vi "Read growables.vi"(9 "Diagram in":refnum<class "Diagram.lvclass">) -> (3 "Diagram out":refnum<class "Diagram.lvclass">, 4 "growables":refnum<class "GrowableFunction.lvclass">[](array[class]))   [LabVIEW 2014, in "Diagram.lvclass"]
uses:
  Diagram.lvclass
  GrowableFunction/GrowableFunction.lvclass
  Diagram.lvclass/Diagram.ctl
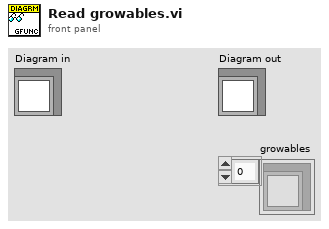
[diagram p1: front panel]
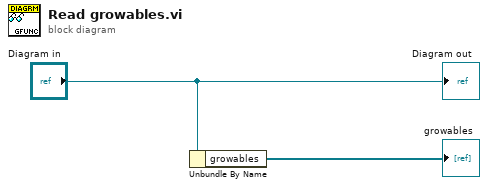
[diagram p0: block diagram]
diagram:
  n1 = Unbundle By Name("Diagram in") -> ("growables"=→"growables":refnum<class "GrowableFunction.lvclass">[])
  "Diagram out" <- "Diagram in"
